vi "Practica1_Introduccion.vi"() -> ()   [LabVIEW 2022 SP3]
panel:
  out "A = B":bool
  out "A < B":bool
  out "A > B":bool
  out "A / B":dbl
  out "A * B":dbl
  out "A - B":dbl
  out "A + B":dbl
  in  "EntradaB":dbl
  in  "EntradaA":dbl
  # "Anahí Montserrat Vázquez Padilla \nPráctica 01: Introducción\n24/01/2024"
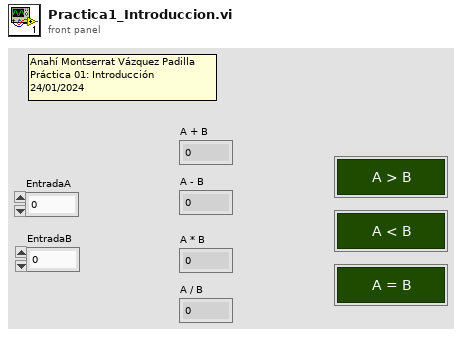
[diagram p1: front panel]
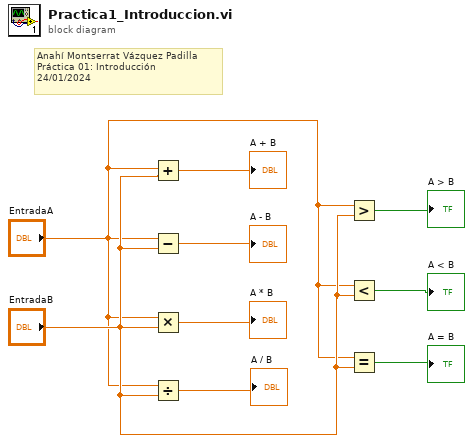
[diagram p0: block diagram]
diagram:
  # "Anahí Montserrat Vázquez Padilla \nPráctica 01: Introducción\n24/01/2024"
  n1 = Add(x="EntradaA", y="EntradaB") -> (x+y=→"A + B":dbl)
  n2 = Subtract(x="EntradaA", y="EntradaB") -> (x-y=→"A - B":dbl)
  n3 = Multiply(x="EntradaA", y="EntradaB") -> (x*y=→"A * B":dbl)
  n4 = Divide(x="EntradaA", y="EntradaB") -> (x/y=→"A / B":dbl)
  n5 = Greater?(x="EntradaA", y="EntradaB") -> (0:→"A > B":bool)
  n6 = Less?(x="EntradaA", y="EntradaB") -> (x < y?=→"A < B":bool)
  n7 = Equal?(x="EntradaA", y="EntradaB") -> (x = y?=→"A = B":bool)
